vi "Read Configuration.vi"(7 "INI Fomatted Cluster Type":variant, 8 "error in (no error)":errorcluster, 11 "Configuration in":refnum<class "Configuration.lvclass">) -> (0 "error out":errorcluster, 2 "Configuration":variant, 3 "Configuration out":refnum<class "Configuration.lvclass">)   [LabVIEW 2019, in "Configuration.lvclass"]
uses:
  Configuration.lvclass
  Configuration.lvclass/Configuration.ctl
  <vilib>/Utility/config.llb/NI_LVConfig.lvlib
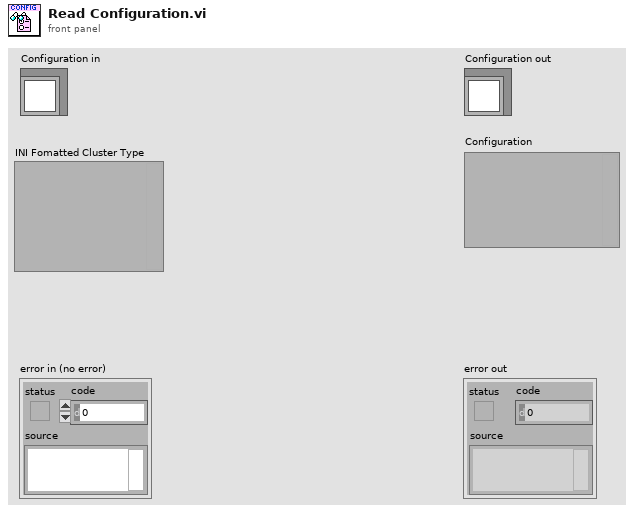
[diagram p1: front panel]
types:
  T1 = typedef "NI_LVConfig.lvlib/Config Data RefNum.ctl" = refnum<k1>
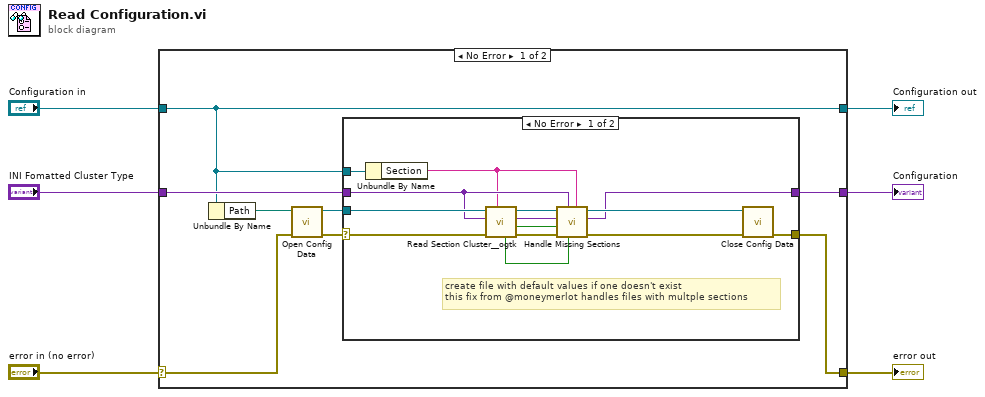
[diagram p0: block diagram]
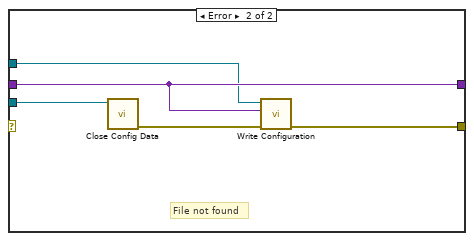
[diagram p2: hidden frame]
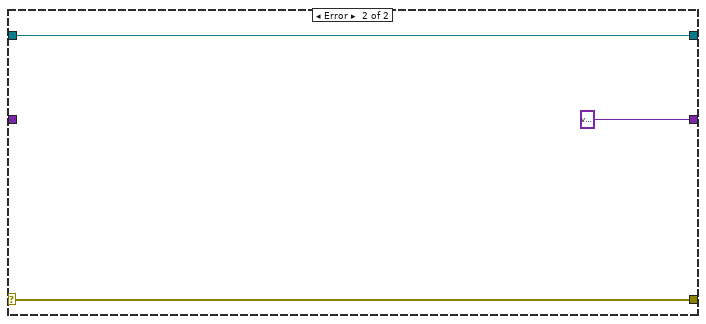
[diagram p3: hidden frame]
diagram:
  n1 = case shown="No Error" "error in (no error)" {
    selector: "error in (no error)" -> [w7 w36]
    tunnel: [w13 w36] -> w1
    tunnel: [w8 w35] -> w6
    tunnel: "Configuration in" -> [w8 w35]
    tunnel: [w12 variant ("Variant")] -> w2
    tunnel: "INI Fomatted Cluster Type" -> [w10 _]
    frame No Error {
      n2 = Unbundle By Name(w8) -> ("Path"=w9:path)
      n3 = call <vilib>:"Open Config Data.vi"("error in (no error)"=w7, "configuration file path"=w9) -> ("error out"=w11:errorcluster, "refnum"=w14:T1)  [unwired: 7 in, 1 out]
      n4 = case shown="No Error" w11 {
        selector: w11 -> [w17 _]
        tunnel: w14 -> [w28 w31]
        tunnel: [w27 w33] -> w13
        tunnel: w10 -> [w25 w32]
        tunnel: [w18 w32] -> w12
        tunnel: w8 -> [w16 w29]
        frame No Error {
          # "create file with default values if one doesn't exist\nthis fix from @moneymerlot handles files with multple sections"
          n5 = Unbundle By Name(w16) -> ("Section"=w15:string)
          n6 = call <userlib>:"Read Section Cluster__ogtk.vi"("section (optional)"=w15, "error in (no error)"=w17, "Section Formatted Cluster Type"=w25, "refnum"=w28) -> ("error out"=w21:errorcluster, "all found?"=w19:bool, "Section Formatted Cluster"=w26:variant, "dup refnum"=w24:T1, "any found?"=w20:bool)  [unwired: 3 in]
          n7 = call "Handle Missing Sections.vi"("section (optional)"=w15, "any found?"=w20, "Section Formatted Cluster In"=w25, "error in (no error)"=w21, "all found?"=w19, "Section Formatted Cluster in"=w26, "Refnum in"=w24) -> ("error out"=w22:errorcluster, "Section Formatted Cluster out"=w18:variant, "Refnum out"=w23:T1)  [unwired: 2 in]
          n8 = call <vilib>:"Close Config Data.vi"("error in (no error)"=w22, "refnum"=w23) -> ("error out"=w27:errorcluster)  [unwired: 8 in, 1 out]
        }
        frame Error {
          # "File not found"
          n9 = call <vilib>:"Close Config Data.vi"("refnum"=w31) -> ("error out"=w30:errorcluster)  [unwired: 9 in, 1 out]
          n10 = call "Write Configuration.vi"("error in (no error)"=w30, "Variant"=w32, "Configuration in"=w29) -> ("error out"=w33:errorcluster)  [unwired: 7 in, 1 out]
        }
      }
    }
    frame Error {
    }
  }
  "error out" <- w1
  "Configuration out" <- w6
  "Configuration" <- w2
